vi "Create_RFID_Baseband v2.vi"(0 "RFID":bool, 5 "Parameters Symbols":T4={"Tari"=8e-06, "PW"=0.5, "factor for \"1\" symbol"=0.5, "RTcal"=2.5, "TRcal"=3.0, "Delimiter"=1.25e-05} {"TRcal" min=1.1 max=3.0 step=0.1; "RTcal" min=2.5 max=3.0 step=0.1; "factor for \"1\" symbol" min=0.5 max=1.0 step=0.1; "PW" min=0.265 max=0.525 step=0.001; "Tari" format="%#_3p"}, 7 "Parameters Select":T3={"Target"=0, "Action"=0, "MemBank"=1, "truncate"=FALSE} {"MemBank" items=["00 RFU", "01 EPC", "10 TID", "11 User"]; "Action" items=["000", "001", "010", "011", "100", "101", "110", "111"]; "Target" items=["000 Inventoried (S0)", "001 Inventoried (S1)", "010 Inventoried (S2)", "011 Inventoried (S3)", "100 SL", "101 RFU", "110 RFU", "111 RFU"]}, 9 "Symbol Rate [Hz]":dbl, 11 "error in":errorcluster, 12 "Parameters Query":T1={"DR"=FALSE, "M"=1, "TRext (T=Pilot Tone)"=FALSE, "Sel"=1, "Session"=0, "Q"=0, "Target"=FALSE} {"Session" items=["S0", "S1", "S2", "S3"]; "Sel" items=["All", "All2", "~SL", "SL"]; "M" items=["M=1", "M=2", "M=4", "M=8"]}) -> (6 "complex waveform":cluster{"t0":dbl, "dt":dbl, "Y":cdb[]}, 15 "error out":errorcluster)   [LabVIEW 2015]
uses:
  <vilib>/addons/Modulation/Analog/support/mod_Set Error Source.vi
  <vilib>/addons/Modulation/Digital/General/MT Generate ASK system parameters (M).vi
  <vilib>/addons/Modulation/Digital/Support/Common/Validators/mod_Generate Filter Coefficients Validate.vi
  <vilib>/addons/Modulation/Digital/General/subVIs/mod_Generate Filter Coefficients.vi
  <vilib>/addons/Modulation/niDMT.lvlib
panel:
  out "ASK system parameters":T2 {"symbol map" format="%.3f"}
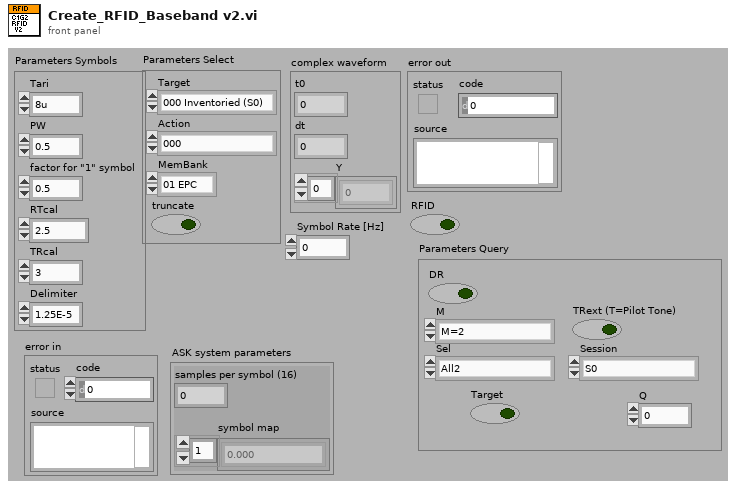
[diagram p1: front panel]
types:
  T1 = cluster{"DR":bool, "M":u16, "TRext (T=Pilot Tone)":bool, "Sel":u16, "Session":u16, "Q":u8, "Target":bool}
  T2 = cluster{"samples per symbol (16)":i32, "symbol map":cdb[]}
  T3 = cluster{"Target":u16, "Action":u16, "MemBank":u16, "truncate":bool}
  T4 = cluster{"Tari":dbl, "PW":dbl, "factor for \"1\" symbol":dbl, "RTcal":dbl, "TRcal":dbl, "Delimiter":dbl}
  T5 = enum16{"none", "Raised Cosine", "Root Raised Cos", "Gaussian"}
  T6 = typedef "niAMT.lvlib/Complex Data Waveform.ctl" = cluster{"t0":dbl, "dt":dbl, "Y":cdb[]}
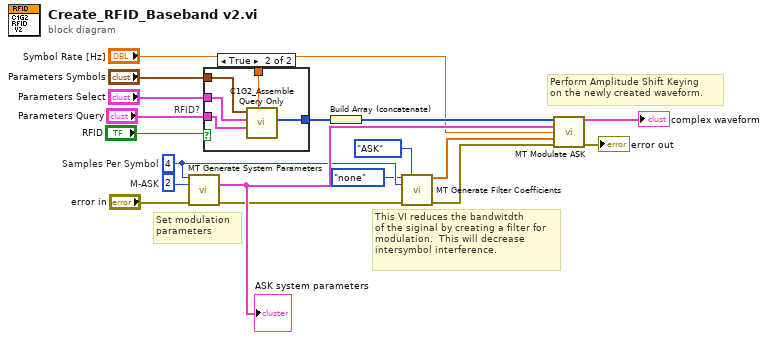
[diagram p0: block diagram]
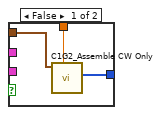
[diagram p2: hidden frame]
diagram:
  w13 = 2  # M-ASK
  w9 = 4  # Samples Per Symbol
  # "Set modulation \nparameters"
  # "Perform Amplitude Shift Keying \non the newly created waveform."
  # "This VI reduces the bandwitdth\nof the siginal by creating a filter for\nmodulation.  This will decrease\nintersymbol interference."
  n1 = call-poly <vilib>:"MT Generate System Parameters.vi"("samples per symbol (16)"=w9, "M-ASK (2)"=w13, "error in (no error)"="error in") -> ("ASK system parameters"=w14:T2, "error out"=w11:errorcluster)  [unwired: 10 in, 1 out]
  "ASK system parameters" <- w14
  n2 = case "RFID?" shown="True" "RFID" {
    tunnel: [w21 w26] -> w6
    tunnel: "Parameters Symbols" -> [w19 w23]
    tunnel: "Parameters Select" -> [_ w24]
    tunnel: "Parameters Query" -> [_ w25]
    tunnel: "Symbol Rate [Hz]" -> [w20 w22]
    frame False {
      n3 = call "C1G2_Assemble CW Only.vi"("Symbol Rate"=w20, "Parameters Symbols"=w19) -> ("Signal out"=w21:u8[])  [unwired: 9 in]
    }
    frame True {
      n4 = call "C1G2_Assemble Query Only.vi"("Symbol Rate"=w22, "Parameters Query"=w25, "Parameters Select"=w24, "Parameters Symbols"=w23) -> ("Signal out"=w26:u8[])  [unwired: 7 in]
    }
  }
  n5 = Build Array (concatenate)(w6) -> (w7:u8[])
  n6 = call <vilib>:"MT Generate Filter Coefficients.vi"("pulse shaping filter (none)"=T5."none", "modulation type"=enum16{"FSK", "PSK", "QAM", "MSK", "PAM", "ASK"}."ASK", "pulse shaping samples per symbol (16)"=w9, "error in (no error)"=w11) -> ("pulse shaping filter coefficients"=w15:dbl[], "error out"=w10:errorcluster)  [unwired: 9 in, 1 out]
  n7 = call <vilib>:"MT Modulate ASK.vi"("input bit stream"=w7, "ASK system parameters"=w14, "symbol rate (Hz)"="Symbol Rate [Hz]", "pulse shaping filter coefficients"=w15, "error in (no error)"=w10) -> ("output complex waveform"=→"complex waveform":T6, "error out"=→"error out":errorcluster)  [unwired: 8 in, 1 out]
